vi "user32_SendMessage.vi"(5 "IParam":u32, 7 "wParam":u32, 8 "error in (no error)":errorcluster, 10 "Msg":u32, 11 "hWnd":u32) -> (0 "error out":errorcluster, 3 "Return Value":u32)   [LabVIEW 2020]
uses:
  user32.dll
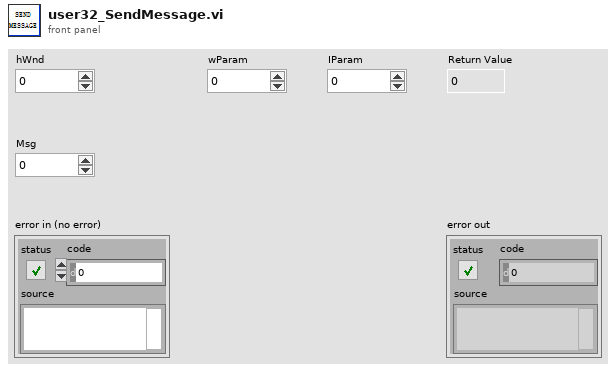
[diagram p1: front panel]
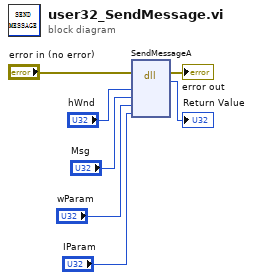
[diagram p0: block diagram]
diagram:
  n1 = dll-call lib="user32.dll" fn="SendMessageA"(error in="error in (no error)", "hWnd"="hWnd", "Msg"="Msg", "wParam"="wParam", "IParam"="IParam") -> (error out=→"error out":errorcluster, "返回值"=→"Return Value":u32)  [unwired: 6 in, 1 out]
